vi "Parse v2.vi"(7 "conversion descriptor":T1 {"conversions"."converted descriptor"."buffer offset" format="%d bytes"; "conversions"."unconverted descriptor"."buffer offset" format="%d bytes"}, 8 "error in (no error)":errorcluster, 9 "converted Buffer":refnum<class "Buffer.lvclass">, 10 "unconverted Buffer":refnum<class "Buffer.lvclass">, 11 "Buffer Converter in":refnum<class "Buffer Converter.lvclass">) -> (0 "error out":errorcluster, 3 "Buffer Converter out":refnum<class "Buffer Converter.lvclass">)   [LabVIEW 2017, in "DSF Core.lvlib" / "Buffer Converter.lvclass"]
uses:
  Buffer Converter.lvclass
  Buffer/Buffer.lvclass
  Type Conversion Descriptor.ctl
  Type Conversion.ctl
  Channel Descriptor.ctl
  DSF Configuration API/Public/Controls/DSF Data Type.ctl
  Buffer/Read Buffer String.vi
  Buffer/Write Buffer String.vi
  DSF Core.lvlib
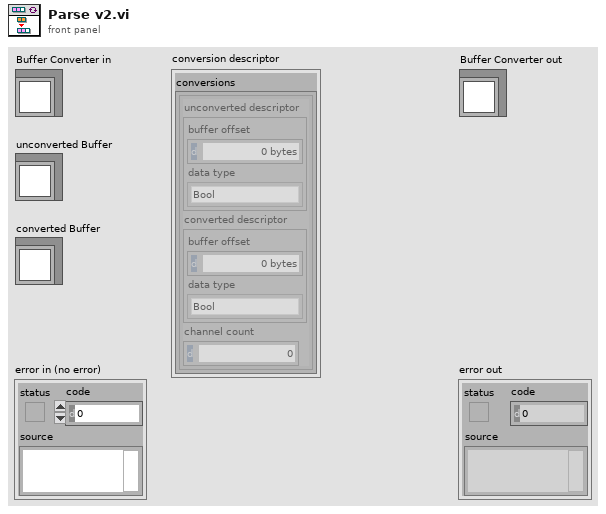
[diagram p1: front panel]
types:
  T1 = typedef "DSF Core.lvlib/Buffer Converter.lvclass/Type Conversion Descriptor.ctl" = cluster{"conversions":T2[]}
  T2 = typedef "DSF Core.lvlib/Buffer Converter.lvclass/Type Conversion.ctl" = cluster{"unconverted descriptor":T3, "converted descriptor":T3, "channel count":u64}
  T3 = typedef "DSF Core.lvlib/Buffer.lvclass/Channel Descriptor.ctl" = cluster{"buffer offset":u64, "data type":T4}
  T4 = typedef "DSF Core.lvlib/DSF Data Type.ctl" = enum8{"Bool", "SGL", "DBL", "I8", "I16", "I32", "I64", "U8", "U16", "U32", "U64"}
  T5 = enum16{"big-endian, network order", "native, host order", "little-endian"}
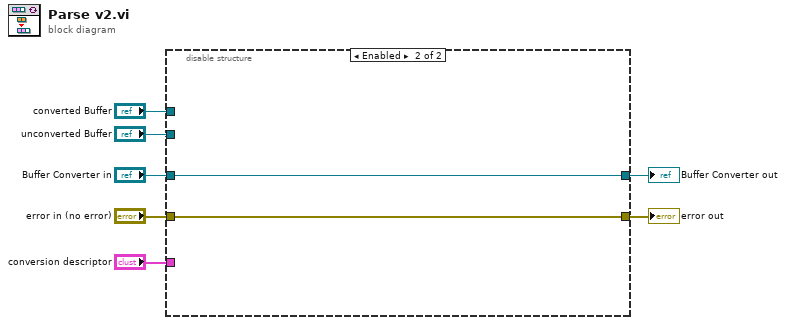
[diagram p0: block diagram]
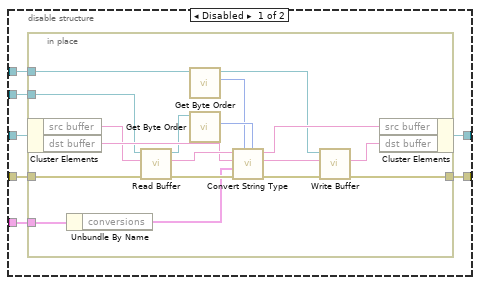
[diagram p2: hidden frame]
diagram:
  n1 = disable-structure shown="Enabled" {
    disable-tunnel: "unconverted Buffer" -> [w14 _]
    disable-tunnel: "converted Buffer" -> [w13 _]
    disable-tunnel: [w12 w33] -> w5
    disable-tunnel: "error in (no error)" -> [w11 w33]
    disable-tunnel: "Buffer Converter in" -> [w10 w34]
    disable-tunnel: [w9 w34] -> w2
    disable-tunnel: "conversion descriptor" -> [w8 _]
    frame Disabled {
      n2 = in-place {
        in-place-border: w14 -> [w19]
        in-place-border: w13 -> [w23]
        in-place-border: [w31] -> w12
        in-place-border: w11 -> [w29]
        in-place-border: w8 -> [w24]
        n3 = in-place-cluster #1(w10) -> ("src buffer"=w21:string, "dst buffer"=w27:string)
        n4 = Unbundle By Name(w24) -> ("conversions"=w16:T2[])
        n5 = call-poly "Read Buffer.vi"("error in (no error)"=w29, "dst string in"=w21, "Buffer in"=w19) -> ("error out"=w30:errorcluster, "dst string out"=w28:string, "Buffer out"=w20:refnum<class "Buffer.lvclass">)  [unwired: 5 in, 1 out]
        n6 = call "Get Byte Order.vi"("Buffer in"=w23) -> ("byte order"=w18:T5, "Buffer out"=w17:refnum<class "Buffer.lvclass">)  [unwired: 9 in]
        n7 = call "Get Byte Order.vi"("Buffer in"=w20) -> ("byte order"=w22:T5)  [unwired: 9 in, 1 out]
        n8 = call "Convert String Type.vi"("src byte order"=w22, "dst byte order"=w18, "error in (no error)"=w30, "conversions"=w16, "dst buffer in"=w27, "src buffer in"=w28) -> ("error out"=w32:errorcluster, "dst buffer out"=w25:string, "src buffer out"=w26:string)  [unwired: 3 in]
        n9 = call-poly "Write Buffer.vi"("error in (no error)"=w32, "src string in"=w25, "Buffer in"=w17) -> ("error out"=w31:errorcluster, "src string out"=w15:string)  [unwired: 5 in, 2 out]
        n10 = in-place-cluster #1("src buffer"=w26, "dst buffer"=w15) -> (w9:refnum<class "Buffer Converter.lvclass">)
      }
    }
    frame Enabled {
    }
  }
  "error out" <- w5
  "Buffer Converter out" <- w2
